vi "Get Serial Number.vi"(8 "error in (no error)":errorcluster, 10 "lpszSerialNum":u8[](array[numeric])=array[4097 elements], 11 "nSensorIP":u32) -> (0 "error out":errorcluster, 2 "lpszSerialNum out":u8[](array[numeric]), 3 "function return":i32)   [LabVIEW 2022 SP3, in "BonTechDetector.lvlib"]
doc: "extern \"C\" BONTECHLIBRARY_API LPTSTR __stdcall GetSerialNumber(unsigned int nSensorIP, LPTSTR lpszSerialNum);\n\nextern \"C\" BONTECHLIBRARY_API int __stdcall GetSerialNumber(unsigned int nSensorIP, LPTSTR lpszSerialNum);"
uses:
  BonTechDetector.lvlib
  C:/Users/Sandeep/Downloads/The Oracle-lv2021/Image Acquisition/Child Classes/BonTechFlatPanel/BonTechWrapperLibrary.dll
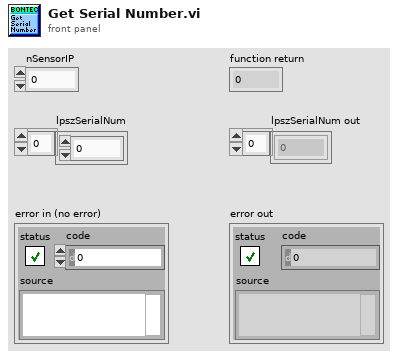
[diagram p1: front panel]
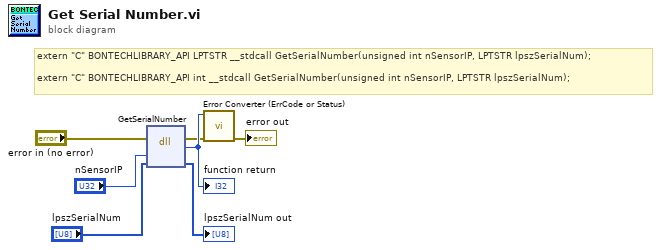
[diagram p0: block diagram]
diagram:
  # "extern \"C\" BONTECHLIBRARY_API LPTSTR __stdcall GetSerialNumber(unsigned int nSensorIP, LPTSTR lpszSerialNum);\n\nextern \"C\" BONTECHLIBRARY_API int __stdcall GetSerialNumber(unsigned int nSensorIP, LPTSTR lpszSerialNum);"
  n1 = dll-call lib="C:/Users/Sandeep/Downloads/The Oracle-lv2021/Image Acquisition/Child Classes/BonTechFlatPanel/BonTechWrapperLibrary.dll" fn="GetSerialNumber"(error in="error in (no error)", "nSensorIP"="nSensorIP", "lpszSerialNum"="lpszSerialNum") -> (error out=w2:errorcluster, "return type"=w7:i32, "lpszSerialNum"=→"lpszSerialNum out":u8[])  [unwired: 3 in, 1 out]
  "function return" <- w7
  n2 = call "Error Converter (ErrCode or Status).vi"("error in (no error)"=w2, "error code"=w7) -> ("error out"=→"error out":errorcluster)  [unwired: 9 in]
